vi "CRYPIC Get New DataView TitleName.vi"() -> (1 "sData_Out":string)   [LabVIEW 2013]
uses:
  CRYMain Sub Window Global.vi
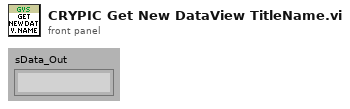
[diagram p1: front panel]
types:
  T1 = typedef "LVRectTypeDef.ctl" = cluster{"Left":i16, "Top":i16, "Right":i16, "Bottom":i16}
  T2 = cluster{"nID":i32[], "Frame":cluster{"nType":i32, "nParent":i32, "pVIW":refnum<vi>, "pSPW":refnum<vi>, "nTypeF":i32, "pVIF":refnum<vi>, "pSPF":refnum<vi>, "nIDSpliter":i32, "nProperty":i32, "Bound":T1, "nID":i32, "nData":i32, "sData":string, "pWVI":refnum<vi>, "sTitle":string, "cPages":cluster{"nPage":i32, "sTitle":string, "sIcon":string, "pVI":refnum<vi>, "nID":i32}[], "pTab":refnum<vi>, "nIDPages":i32[], "pSPT":refnum<vi>, "sTemp":string, "nDockID":i32, "nDockLR":i32, "sIcon":string}[]}
  T3 = cluster{"nType":i32, "nParent":i32, "pVIW":refnum<vi>, "pSPW":refnum<vi>, "nTypeF":i32, "pVIF":refnum<vi>, "pSPF":refnum<vi>, "nIDSpliter":i32, "nProperty":i32, "Bound":T1, "nID":i32, "nData":i32, "sData":string, "pWVI":refnum<vi>, "sTitle":string, "cPages":cluster{"nPage":i32, "sTitle":string, "sIcon":string, "pVI":refnum<vi>, "nID":i32}[], "pTab":refnum<vi>, "nIDPages":i32[], "pSPT":refnum<vi>, "sTemp":string, "nDockID":i32, "nDockLR":i32, "sIcon":string}[]
  T4 = enum16{"OK", "Yes", "YesNo", "YesNoCancel", "ReplaceAppend"}
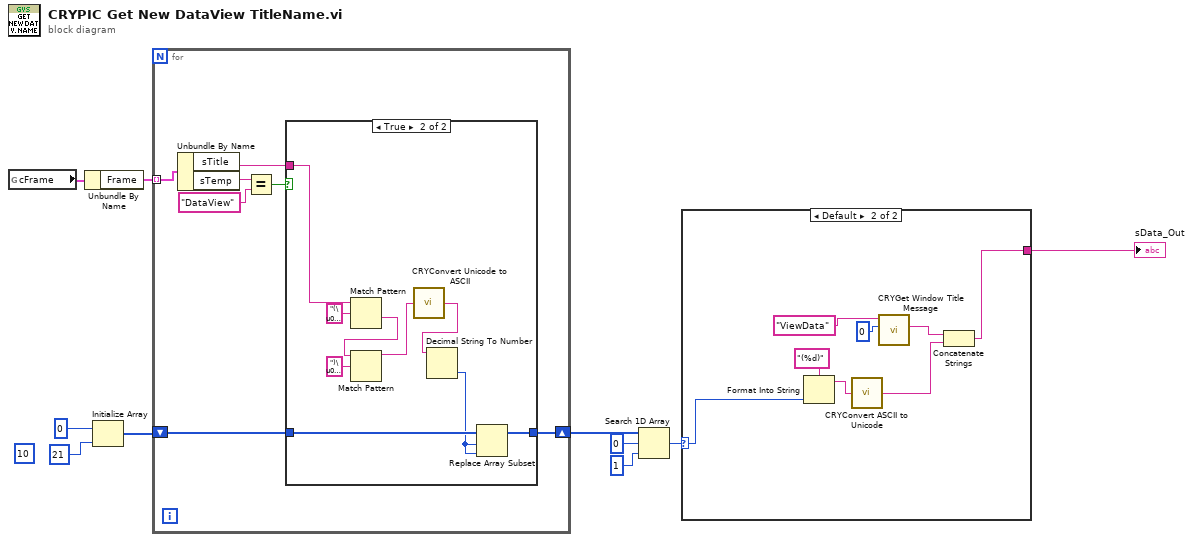
[diagram p0: block diagram]
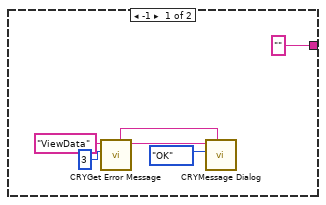
[diagram p2: hidden frame]
diagram:
  (unwired) 10 ("dimension size")
  n1 = global read "CRYMain Sub Window Global.vi" "cFrame"() -> (w10:T2)
  n2 = Unbundle By Name(w10) -> ("Frame"=w9:T3)
  n3 = Initialize Array(0, 21 ("dimension size")) -> (w6:i32[])
  n4 = for {
    tunnel: w9 -> [w17] mode=indexing
    shift-right: [w11] -> w5
    shift-left: w6 -> [w12]
    n5 = Unbundle By Name(w17) -> ("sTitle"=w13:string, "sTemp"=w14:string)
    n6 = Equal?(x=w14, y="DataView") -> (x = y?=w15:bool)
    n7 = case shown="True" w15 {
      tunnel: w13 -> [_ w24]
      tunnel: w12 -> [w18 w22]
      tunnel: [w18 w23] -> w11
      frame False {
      }
      frame True {
        n8 = Match Pattern(string=w24, regular expression="(\u0000") -> (after substring=w27:string)  [unwired: 1 in, 3 out]
        n9 = Match Pattern(string=w27, regular expression=")\u0000") -> (before substring=w20:string)  [unwired: 1 in, 3 out]
        n10 = call "CRYConvert Unicode to ASCII.vi"("Unicode"=w20) -> ("ASCII"=w19:string)  [unwired: 4 in]
        n11 = Decimal String To Number(string=w19) -> (number=w21:i32)  [unwired: 2 in, 1 out]
        n12 = Replace Array Subset(array=w22, new element=w21, index=w21) -> (w23:i32[])
      }
    }
  }
  n13 = Search 1D Array(1D array=w5, element=0, start index (0)=1) -> (index of element=w2:i32)
  n14 = case shown="Default" w2 {
    selector: w2 -> [_ w35]
    tunnel: ["" w34] -> w1
    frame -1 {
      n15 = call "CRYGet Error Message.vi"("Error No"=3, "Kind"="ViewData") -> ("Message"=w28:string, "Window Title"=w29:string)  [unwired: 4 in, 4 out]
      n16 = call "CRYMessage Dialog.vi"("Window Title"=w29, "YesNoCancel"=T4."OK", "Message Content"=w28) -> ()  [unwired: 7 in, 2 out]
    }
    frame Default {
      n17 = Format Into String(format string="(%d)", w35) -> (resulting string=w39:string)  [unwired: 2 in, 1 out]
      n18 = call "CRYConvert ASCII to Unicode.vi"("ASCII"=w39) -> ("Unicode"=w41:string)  [unwired: 4 in]
      n19 = call "CRYGet Window Title Message.vi"("No"=0 ("Error No"), "Kind"="ViewData") -> ("Unicode String"=w40:string)  [unwired: 4 in, 5 out]
      n20 = Concatenate Strings(w40, w41) -> (w34:string)
    }
  }
  "sData_Out" <- w1
